vi "RemoveDataListener.vi"(8 "error in (no error)":errorcluster, 10 "Label":string, 11 "GRMActor in":refnum<class "GeneralRMActor.lvclass">) -> (0 "error out":errorcluster, 2 "key not found?":bool, 3 "GRMActor out":refnum<class "GeneralRMActor.lvclass">)   [LabVIEW 2020, in "GeneralRMActor.lvlib" / "GeneralRMActor.lvclass"]
uses:
  GeneralRMActor.lvclass
  GeneralRMActor.lvclass/GeneralRMActor.ctl
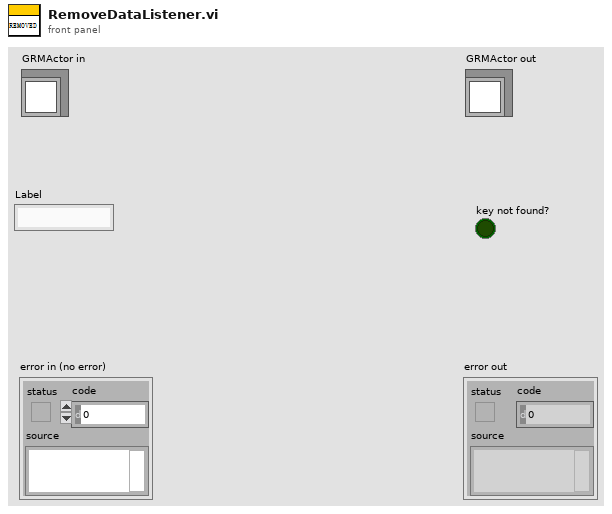
[diagram p1: front panel]
types:
  T1 = map{string, refnum<class "Message Enqueuer.lvclass">}
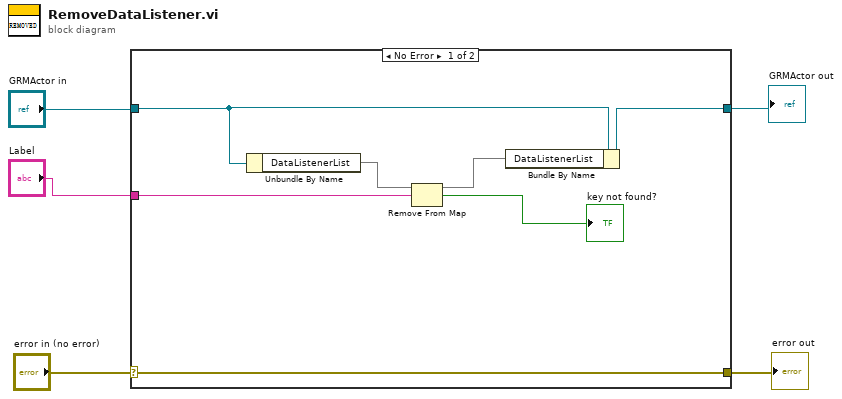
[diagram p0: block diagram]
diagram:
  n1 = case shown="No Error" "error in (no error)" {
    selector: "error in (no error)" -> [w12 w14]
    tunnel: [w12 w14] -> w3
    tunnel: [w9 w13] -> w4
    tunnel: "GRMActor in" -> [w11 w13]
    tunnel: "Label" -> [w7 _]
    frame No Error {
      n2 = Unbundle By Name(w11) -> ("DataListenerList"=w10:T1)
      n3 = Remove From Map(10:w7, 11:w10) -> (2:→"key not found?":bool, 3:w8:T1)  [unwired: 1 out]
      n4 = Bundle By Name(cluster=w11, "DataListenerList"=w8) -> (w9:refnum<class "GeneralRMActor.lvclass">)
    }
    frame Error {
    }
  }
  "error out" <- w3
  "GRMActor out" <- w4
